vi "test Encode and Decode - Discretes Only.vi"(8 "error in (no error)":errorcluster, 11 "TestCase in":refnum<class "AIM ARINC 664 EncodeDecode.lvclass">) -> (0 "error out":errorcluster, 3 "TestCase out":refnum<class "AIM ARINC 664 EncodeDecode.lvclass">)   [LabVIEW 2020, in "AIM ARINC 664 EncodeDecode.lvclass"]
uses:
  AIM ARINC 664 EncodeDecode.lvclass
  Shared/Encoding (Arinc664).ctl
  <vilib>/addons/_JKI Toolkits/VI Tester/TestCase.llb/TestCase.lvclass
  C:/Program Files/National Instruments/LabVIEW 2024/vi.lib/addons/_JKI Toolkits/VI Tester/TestCase.llb/TestCase.lvclass
panel:
  out "index of first error":i32
  out "Parameters":T2(array[cluster]) {"encoding" items=["BNR", "BCD", "Discrete", "Signed_32", "Signed_64", "Float_32", "Float_64", "Opaque"]}
  in  "number of discretes":i32=512
  out "Result array out":bool[](array[boolean])
  out "Values in":dbl[](array[numeric])
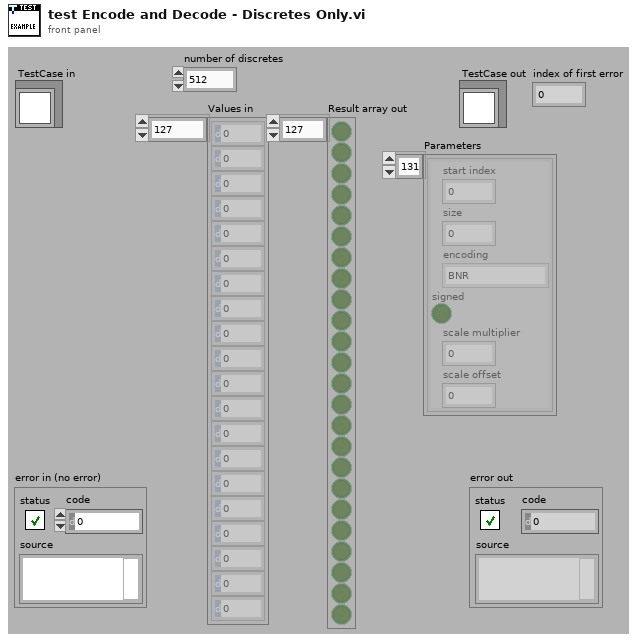
[diagram p1: front panel]
types:
  T1 = typedef "Encoding (Arinc664).ctl" = u16
  T2 = cluster{"start index":i32, "size":i32, "encoding":T1, "signed":bool, "scale multiplier":dbl, "scale offset":dbl}[]
  T3 = cluster{"start index":i32, "size":i32, "encoding":T1, "signed":bool, "scale multiplier":dbl, "scale offset":dbl}
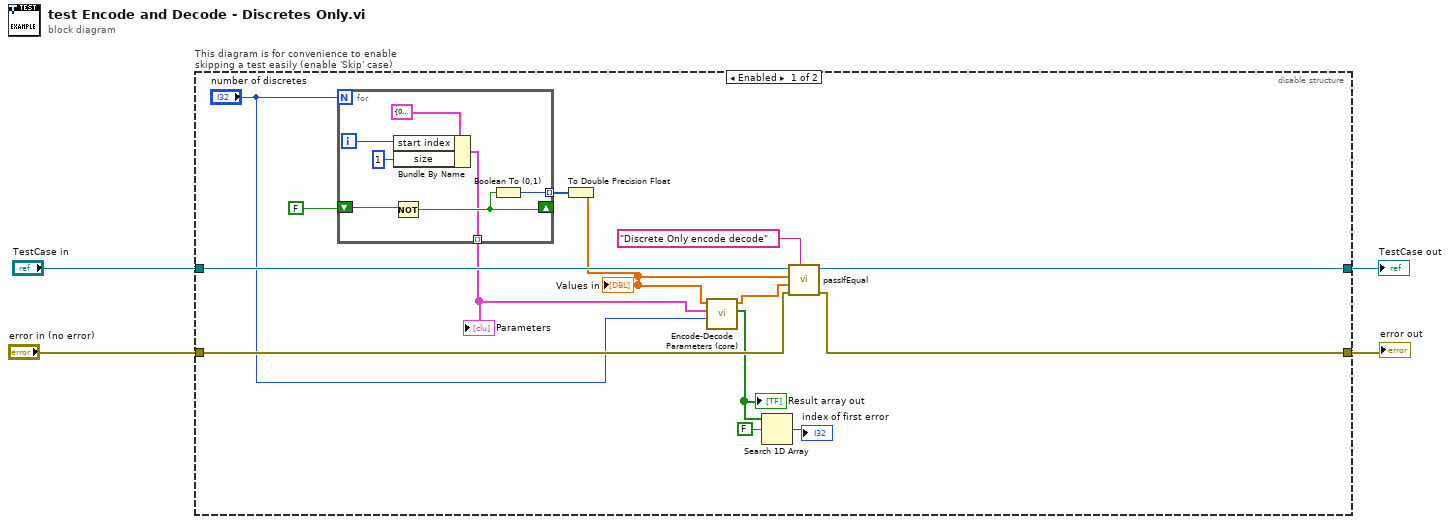
[diagram p0: block diagram]
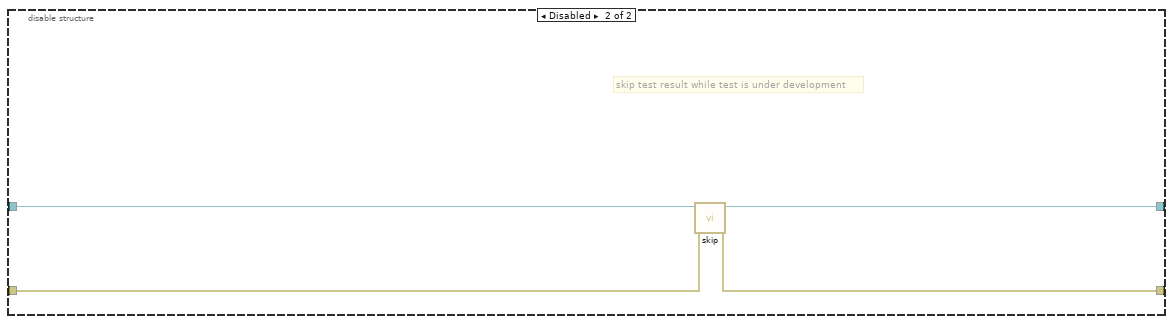
[diagram p2: hidden frame]
diagram:
  n1 = disable-structure "This diagram is for convenience to enable skipping a test easily (enable 'Skip' case)" shown="Enabled" {
    disable-tunnel: "TestCase in" -> [w18 w29]
    disable-tunnel: [w15 w27] -> w1
    disable-tunnel: [w16 w28] -> w3
    disable-tunnel: "error in (no error)" -> [w17 w26]
    frame Enabled {
      n2 = for {
        N: "number of discretes" -> [_]
        shift-right: [w23] -> _
        shift-left: FALSE -> [w24]
        tunnel: [w22] -> w10 mode=indexing
        tunnel: [w21] -> w11 mode=indexing
        i -> [w20]
        n3 = Not(x=w24) -> (.not. x?=w23:bool)
        n4 = Bundle By Name(cluster=T3 {"start index"=0, "size"=64, "encoding"=2, "signed"=TRUE, "scale multiplier"=1.0, "scale offset"=0.0} ("Parameters 2"), "start index"=w20, "size"=1) -> (w21:T3)
        n5 = Boolean To (0,1)(Boolean=w23) -> (0, 1=w22:i16)
      }
      "Parameters" <- w11
      n6 = To Double Precision Float(number=w10) -> (double precision float=w9:dbl[])
      "Values in" <- w9
      n7 = call "Encode-Decode Parameters (core).vi"("Payload size - bytes"="number of discretes", "Parameters"=w11, "Values in"=w9) -> ("Result array out"=w8:bool[], "Values out"=w13:dbl[])  [unwired: 7 in]
      "Result array out" <- w8
      n8 = Search 1D Array(1D array=w8, element=FALSE) -> (index of element=→"index of first error":i32)  [unwired: 1 in]
      n9 = call-dynamic "passIfEqual.vi"("custom report message (\"\")"="Discrete Only encode decode" ("custom report message (\"\")"), "error in (no error)"=w17, "y"=w13, "x"=w9, "TestCase in"=w18) -> ("error out"=w16:errorcluster, "TestCase out"=w15:refnum<class "AIM ARINC 664 EncodeDecode.lvclass">)  [unwired: 5 in]
    }
    frame Disabled {
      # "skip test result while test is under development"
      n10 = call <vilib>:"skip.vi"("error in (no error)"=w26, "TestCase in"=w29) -> ("error out"=w28:errorcluster, "TestCase out"=w27:refnum<class "AIM ARINC 664 EncodeDecode.lvclass">)  [unwired: 8 in]
    }
  }
  "error out" <- w3
  "TestCase out" <- w1
